vi "Spatio Plot - PDF.vi"(11 "Data Cluster":T6={"Selected File"=path "", "Full Text File"=[], "Data Array"=[], "Times Array"=[], "Sensor Array"=[], "Subset Array"=[], "Smoothness Values"=[], "Sensor Select 1"=refnum, "Sensor Select 2"=refnum, "Sensor Select 3"=refnum, "Sensor Select 4"=refnum, "Start Times"=[], "End Times"=[], "Cursor List"=[{"Name"="Event Marker          ", "Color"=16777200, "Style"=0, "Point Style"=0, "Name Visible"=FALSE, "Allow Drag"=FALSE, "Cursor Mode"=0, "Plot"=0, "Index"=0, "Position"={"X"=4.0, "Y"=1.0}, "X Scale"=0, "Y Scale"=0, "Watch Plots"=[], "Watch All Plots"=FALSE, "Plot Area"=0, "Label Offset"={"X"=-50.0, "Y"=150.0}}, {"Name"="Upper Sensor", "Color"=13816500, "Style"=6, "Point Style"=0, "Name Visible"=FALSE, "Allow Drag"=FALSE, "Cursor Mode"=0, "Plot"=0, "Index"=0, "Position"={"X"=-1.0, "Y"=5.0}, "X Scale"=0, "Y Scale"=0, "Watch Plots"=[], "Watch All Plots"=FALSE, "Plot Area"=0, "Label Offset"={"X"=0.0, "Y"=0.0}}, {"Name"="Lower Sensor", "Color"=13816500, "Style"=6, "Point Style"=0, "Name Visible"=FALSE, "Allow Drag"=FALSE, "Cursor Mode"=0, "Plot"=0, "Index"=0, "Position"={"X"=-1.0, "Y"=30.0}, "X Scale"=0, "Y Scale"=0, "Watch Plots"=[], "Watch All Plots"=FALSE, "Plot Area"=0, "Label Offset"={"X"=0.0, "Y"=0.0}}], "Listbox 1"=refnum, "Listbox 2"=refnum, "Listbox 3"=refnum, "Listbox 4"=refnum, "Labels"=["Why", "is", "this", "still", "not", "built", "into", "Labview?", "This", "is", "shameful."], "Event Array"=[], "Event Names"=[], "Event Times"=[], "Save Plot Button"=refnum, "Sensor Plot Refs"=[], "Selected Event (Title)"="", "Upper Cursor"=0.0, "Lower Cursor"=0.0, "Z Max"=0.0, "Z Min"=0.0}) -> (3 "cancelled":bool)   [LabVIEW 2020]
uses:
  Controls/DataCluster.ctl
  <vilib>/Utility/miscctls.llb/LVCursorListTypeDef.ctl
  <vilib>/Heliosphere Research LLC/Advanced Plotting Toolkit/api_annotations/HVLineProperties.ctl
  <vilib>/Heliosphere Research LLC/Advanced Plotting Toolkit/properties/Line.ctl
  <vilib>/Heliosphere Research LLC/Advanced Plotting Toolkit/properties/Line_Style.ctl
  <vilib>/Heliosphere Research LLC/Advanced Plotting Toolkit/typedefs/PlotColor.ctl
  <vilib>/Heliosphere Research LLC/Advanced Plotting Toolkit/properties/Display.ctl
  <vilib>/Heliosphere Research LLC/Advanced Plotting Toolkit/api_plotting/ContourRange.ctl
  <vilib>/Heliosphere Research LLC/Advanced Plotting Toolkit/api_annotations/LabelProperties.ctl
  <vilib>/Heliosphere Research LLC/Advanced Plotting Toolkit/properties/Text.ctl
  <vilib>/Heliosphere Research LLC/Advanced Plotting Toolkit/properties/Text_FontSize.ctl
  <vilib>/Heliosphere Research LLC/Advanced Plotting Toolkit/properties/Text_FontStyle.ctl
  <userlib>/_OpenG.lib/array/array.llb/Reverse 2D Array (DBL)__ogtk.vi
  <vilib>/Heliosphere Research LLC/Advanced Plotting Toolkit/api_plotting/ContourFilled_Automatic.vi
  <vilib>/Heliosphere Research LLC/Advanced Plotting Toolkit/Advanced Plotting Toolkit.lvlib
panel:
  in  "Properties":T1={"Line"={"Style"=enum."Automatic", "Color"=2147483647, "Width"=nan}, "Display"={"Alpha"=nan, "Z Order"=nan}} {"Line"."Color" items=["Automatic"=2147483647, "Black"=0, "White"=16777215, "Red"=16711680, "Green"=2263842, "Blue"=255, "Cyan"=65535, "Magenta"=16711935, "Yellow"=16776960]}
  out "Plot":picture
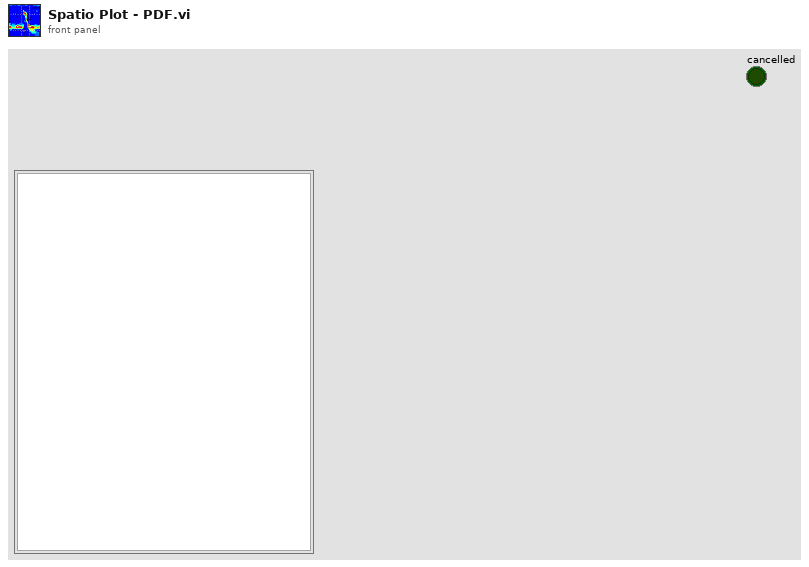
[diagram p1: front panel]
types:
  T1 = typedef "Advanced Plotting Toolkit.lvlib/HVLineProperties.ctl" = cluster{"Line":T2, "Display":T5}
  T2 = typedef "Advanced Plotting Toolkit.lvlib/Line.ctl" = cluster{"Style":T3, "Color":T4, "Width":sgl}
  T3 = typedef "Advanced Plotting Toolkit.lvlib/Line_Style.ctl" = enum16{"Automatic", "Solid", "Dashed", "Dotted", "Dash-dot", "Invisible"}
  T4 = typedef "Advanced Plotting Toolkit.lvlib/PlotColor.ctl" = u32
  T5 = typedef "Advanced Plotting Toolkit.lvlib/Display.ctl" = cluster{"Alpha":dbl, "Z Order":dbl}
  T6 = typedef "DataCluster.ctl" = cluster{"Selected File":path, "Full Text File":string[][], "Data Array":dbl[][], "Times Array":dbl[], "Sensor Array":dbl[], "Subset Array":dbl[][], "Smoothness Values":dbl[], "Sensor Select 1":refnum<vi>, "Sensor Select 2":refnum<vi>, "Sensor Select 3":refnum<vi>, "Sensor Select 4":refnum<vi>, "Start Times":dbl[], "End Times":dbl[], "Cursor List":T7, "Listbox 1":refnum<vi>, "Listbox 2":refnum<vi>, "Listbox 3":refnum<vi>, "Listbox 4":refnum<vi>, "Labels":string[], "Event Array":dbl[][], "Event Names":string[], "Event Times":dbl[], "Save Plot Button":refnum<vi>, "Sensor Plot Refs":refnum<vi>[], "Selected Event (Title)":string, "Upper Cursor":dbl, "Lower Cursor":dbl, "Z Max":dbl, "Z Min":dbl}
  T7 = typedef "LVCursorListTypeDef.ctl" = cluster{"Name":string, "Color":u32, "Style":u8, "Point Style":u8, "Name Visible":bool, "Allow Drag":bool, "Cursor Mode":u32, "Plot":i32, "Index":i32, "Position":cluster{"X":dbl, "Y":dbl}, "X Scale":u32, "Y Scale":u32, "Watch Plots":i32[], "Watch All Plots":bool, "Plot Area":i32, "Label Offset":cluster{"X":dbl, "Y":dbl}}[]
  T8 = typedef "Advanced Plotting Toolkit.lvlib/LabelProperties.ctl" = cluster{"Text":T9}
  T9 = typedef "Advanced Plotting Toolkit.lvlib/Text.ctl" = cluster{"Color":T4, "Background Color":T4, "Font Size (points)":T10, "Font Style":T11, "Rotation Angle":dbl}
  T10 = typedef "Advanced Plotting Toolkit.lvlib/Text_FontSize.ctl" = i32
  T11 = typedef "Advanced Plotting Toolkit.lvlib/Text_FontStyle.ctl" = enum16{"Automatic", "Normal", "Italic", "Bold"}
  T12 = typedef "Advanced Plotting Toolkit.lvlib/ContourRange.ctl" = cluster{"Min Level":dbl, "Max Level":dbl}
  T13 = typedef "Advanced Plotting Toolkit.lvlib/PlotID.ctl" = i32
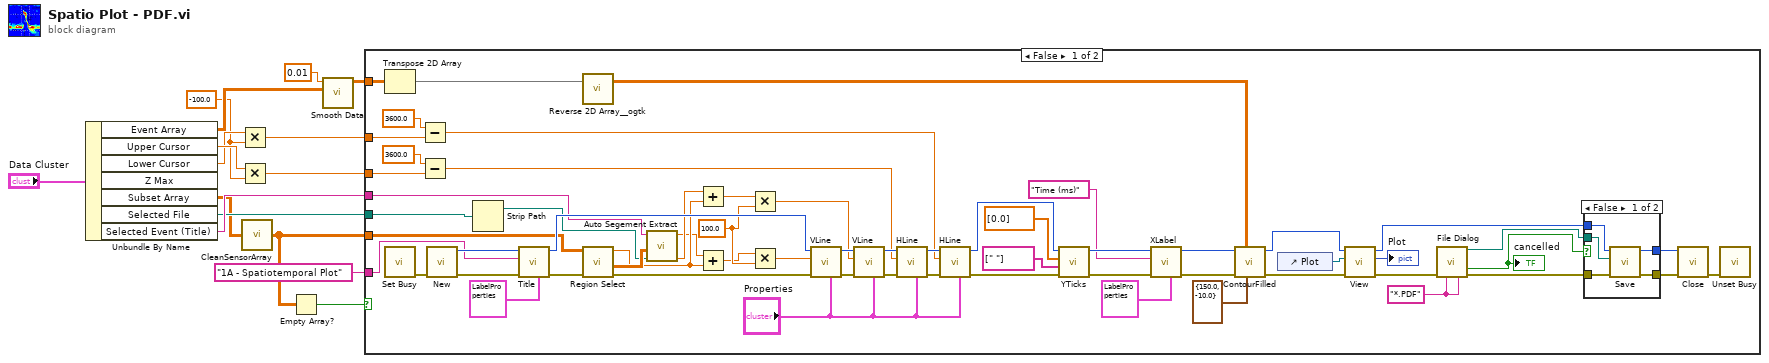
[diagram p0: block diagram]
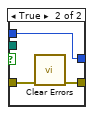
[diagram p2: hidden frame]
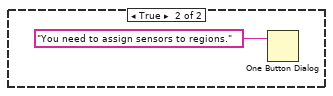
[diagram p3: hidden frame]
diagram:
  w4 = -100.0 ("y")
  n1 = Unbundle By Name("Data Cluster") -> ("Event Array"=w14:dbl[][], "Upper Cursor"=w10:dbl, "Lower Cursor"=w8:dbl, "Subset Array"=w2:dbl[][], "Selected File"=w5:path, "Selected Event (Title)"=w6:string)  [unwired: 1 out]
  n2 = Multiply(x=w8, y=w4) -> (x*y=w7:dbl)
  n3 = Multiply(x=w10, y=w4) -> (x*y=w9:dbl)
  n4 = call "CleanSensorArray.vi"("Sensor Data Array"=w2) -> ("Clean Array"=w1:dbl[][])  [unwired: 4 in]
  n5 = Empty Array?(array=w1) -> (empty?=w3:bool)
  n6 = call "Smooth Data.vi"("Data Array"=w14, "dt"=0.01) -> ("Resampled Array"=w13:dbl[][])  [unwired: 8 in, 1 out]
  n7 = case shown="False" w3 {
    tunnel: w13 -> [w69 _]
    tunnel: "1A - Spatiotemporal Plot" ("Title") -> [w61 _]
    tunnel: w9 -> [w36 _]
    tunnel: w7 -> [w32 _]
    tunnel: w6 -> [w27 _]
    tunnel: w5 -> [w26 _]
    tunnel: w1 -> [w16 _]
    frame False {
      w22 = 100.0 ("y")
      w37 = "*.PDF" ("pattern label")
      n8 = Transpose 2D Array(2D array=w69) -> (transposed array=w68:dbl[][])
      n9 = call <vilib>:"Set Busy.vi"() -> ("error out"=w66:errorcluster)  [unwired: 10 in, 1 out]
      n10 = Subtract(x=3600.0, y=w32) -> (x-y=w31:dbl)
      n11 = Subtract(x=3600.0, y=w36) -> (x-y=w34:dbl)
      n12 = call <vilib>:"New.vi"("error in (no error)"=w66) -> ("error out"=w63:errorcluster, "Plot ID"=w64:T13)  [unwired: 9 in]
      n13 = Strip Path(path=w26) -> (stripped path=w25:path)  [unwired: 1 out]
      n14 = call <vilib>:"Title.vi"("Properties"=T8 {"Text"={"Color"=2147483647, "Background Color"=2147483647, "Font Size (points)"=-4, "Font Style"=enum."Bold", "Rotation Angle"=nan}}, "error in (no error)"=w63, "Title"=w61, "Plot ID"=w64) -> ("error out"=w30:errorcluster, "Plot ID out"=w62:T13)  [unwired: 6 in]
      n15 = call-poly <userlib>:"Reverse 2D Array__ogtk.vi"("Array"=w68) -> ("Reversed Array"=w48:dbl[][])  [unwired: 2 in]
      n16 = call "Region Select.vi"("Error In"=w30, "Sensor Data Array"=w16) -> ("Error Out"=w29:errorcluster, "Trimmed Event"=w28:dbl[][], "Segement Start"=w19:dbl)  [unwired: 7 in]
      n17 = call "Auto Segement Extract.vi"("Save Path"=w25, "Sensor Data Array"=w28, "Title"=w27) -> ("End"=w18:dbl, "Start"=w17:dbl)  [unwired: 1 in, 2 out]
      n18 = Add(x=w18, y=w19) -> (x+y=w21:dbl)
      n19 = Add(x=w17, y=w19) -> (x+y=w20:dbl)
      n20 = Multiply(x=w21, y=w22) -> (x*y=w23:dbl)
      n21 = Multiply(x=w20, y=w22) -> (x*y=w24:dbl)
      n22 = call <vilib>:"VLine.vi"("Properties"="Properties", "error in (no error)"=w29, "X (data coords)"=w24, "Plot ID"=w62) -> ("error out"=w55:errorcluster, "Plot ID Out"=w56:T13)  [unwired: 6 in]
      n23 = call <vilib>:"VLine.vi"("Properties"="Properties", "error in (no error)"=w55, "X (data coords)"=w23, "Plot ID"=w56) -> ("error out"=w54:errorcluster, "Plot ID Out"=w57:T13)  [unwired: 6 in]
      n24 = call <vilib>:"HLine.vi"("Properties"="Properties", "error in (no error)"=w54, "Y (data coords)"=w34, "Plot ID"=w57) -> ("error out"=w59:errorcluster, "Plot ID Out"=w60:T13)  [unwired: 6 in]
      n25 = call <vilib>:"HLine.vi"("Properties"="Properties", "error in (no error)"=w59, "Y (data coords)"=w31, "Plot ID"=w60) -> ("error out"=w51:errorcluster, "Plot ID Out"=w52:T13)  [unwired: 6 in]
      n26 = call <vilib>:"YTicks.vi"("error in (no error)"=w51, "Tick Labels"=string[] [" "], "Tick Locations"=dbl[] [0.0], "Plot ID"=w52) -> ("error out"=w46:errorcluster, "Plot ID Out"=w47:T13)  [unwired: 6 in]
      n27 = call <vilib>:"XLabel.vi"("Properties"=T8 {"Text"={"Color"=2147483647, "Background Color"=2147483647, "Font Size (points)"=-3, "Font Style"=enum."Bold", "Rotation Angle"=nan}}, "error in (no error)"=w46, "Label"="Time (ms)", "Plot ID"=w47) -> ("error out"=w44:errorcluster, "Plot ID out"=w45:T13)  [unwired: 6 in]
      n28 = call-poly <vilib>:"ContourFilled.vi"("Contour Range"=T12 {"Min Level"=150.0, "Max Level"=-10.0}, "Z Data"=w48, "error in (no error)"=w44, "Plot ID"=w45) -> ("error out"=w76:errorcluster, "Plot ID Out"=w71:T13)  [unwired: 6 in]
      n29 = control-ref of="Plot"() -> (w70:refnum<vi>)
      n30 = call <vilib>:"View.vi"("error in (no error)"=w76, "Ref for Sizing"=w70, "Plot ID"=w71) -> ("error out"=w41:errorcluster, "Picture"=→"Plot":picture, "Plot ID Out"=w72:T13)  [unwired: 6 in]
      n31 = call "File Dialog"("error in"=w41, "pattern (all files)"=w37, "pattern label"=w37) -> ("selected path"=w38:path, "cancelled"=w39:bool, "error out"=w40:errorcluster)  [unwired: 9 in, 1 out]
      "cancelled" <- w39
      n32 = case shown="False" w39 {
        tunnel: [w81 w82] -> w74
        tunnel: [w80 w84] -> w73
        tunnel: w72 -> [w79 w84]
        tunnel: w40 -> [w78 w83]
        tunnel: w38 -> [w77 _]
        frame False {
          n33 = call <vilib>:"Save.vi"("error in (no error)"=w78, "Path"=w77, "Plot ID In"=w79) -> ("error out"=w81:errorcluster, "Plot ID Out"=w80:T13)  [unwired: 7 in]
        }
        frame True {
          n34 = call <vilib>:"Clear Errors.vi"("error in (no error)"=w83) -> ("error out"=w82:errorcluster)  [unwired: 5 in, 1 out]
        }
      }
      n35 = call <vilib>:"Close.vi"("error in (no error)"=w74, "Plot ID"=w73) -> ("error out"=w65:errorcluster)  [unwired: 9 in]
      n36 = call <vilib>:"Unset Busy.vi"("error in (no error)"=w65) -> ()  [unwired: 10 in, 1 out]
    }
    frame True {
      n37 = One Button Dialog(message="You need to assign sensors to regions.") -> ()  [unwired: 1 in, 1 out]
    }
  }
